vi "State Entry.vi"(8 "error in (no error)":errorcluster, 11 "View Model":T1) -> (0 "error out":errorcluster, 3 "View Model":T1)   [LabVIEW 2017]
doc: "Start processing ATM controller state when state just appear."
uses:
  View Model/Controls/View Model.ctl
  View Model/Controls/Shared Model.ctl
  Error Handler/Controls/Error Model.ctl
  Error Handler/Controls/Error Data.ctl
  Error Handler/Controls/Error Type.ctl
  Error Handler/Controls/Error Source.ctl
  Configuration/Controls/Config Model.ctl
  Configuration/Controls/Config CMD.ctl
  Configuration/Controls/Config Command.ctl
  Controls/Controller Model.ctl
  Controls/Controller Overhead.ctl
  Controls/Controller Transaction.ctl
  Controls/Controller State.ctl
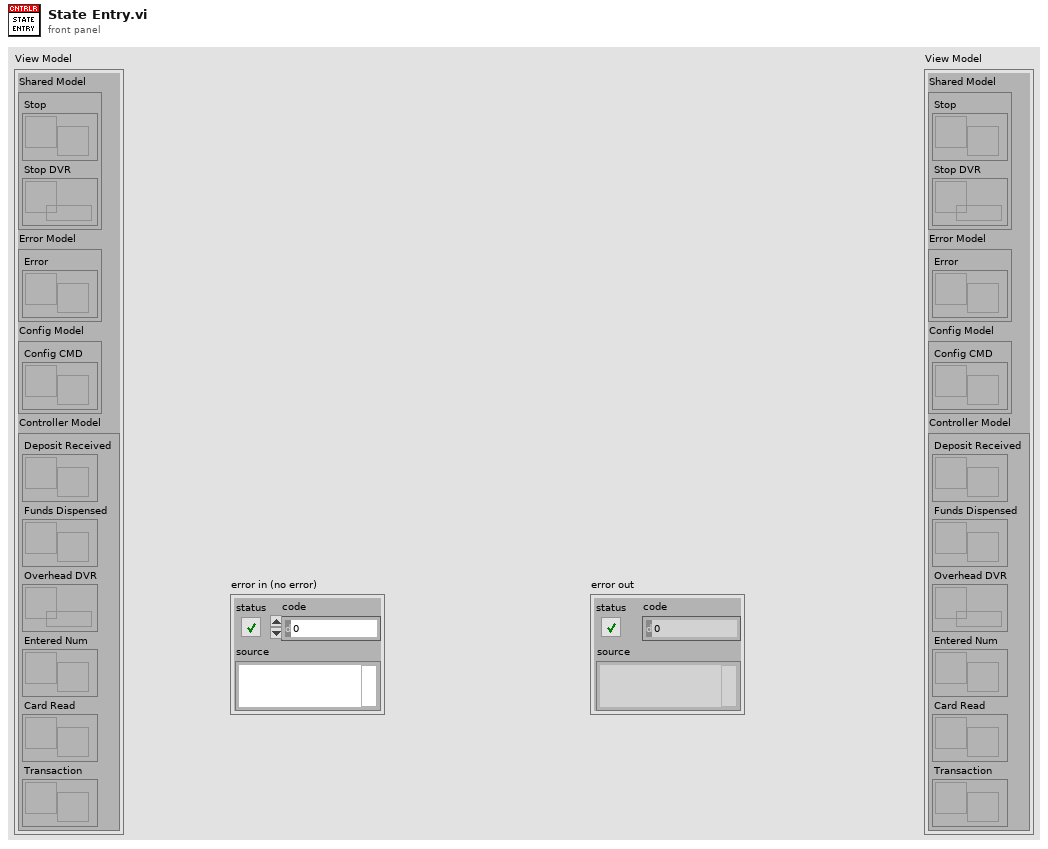
[diagram p1: front panel]
types:
  T1 = typedef "View Model.ctl" = cluster{"Shared Model":T2, "Error Model":T3, "Config Model":T4, "Controller Model":T5}
  T2 = typedef "Shared Model.ctl" = cluster{"Stop":refnum<user-event>, "Stop DVR":refnum<data-value>}
  T3 = typedef "Error Model.ctl" = cluster{"Error":refnum<user-event>}
  T4 = typedef "Config Model.ctl" = cluster{"Config CMD":refnum<user-event>}
  T5 = typedef "Controller Model.ctl" = cluster{"Deposit Received":refnum<user-event>, "Funds Dispensed":refnum<user-event>, "Overhead DVR":refnum<data-value>, "Entered Num":refnum<user-event>, "Card Read":refnum<user-event>, "Transaction":refnum<user-event>}
  T6 = typedef "Controller State.ctl" = enum16{"Idle", "Initial", "Login", "Balance Inquiry", "Deposit", "Withdrawal", "Fast Cash", "Terminate"}
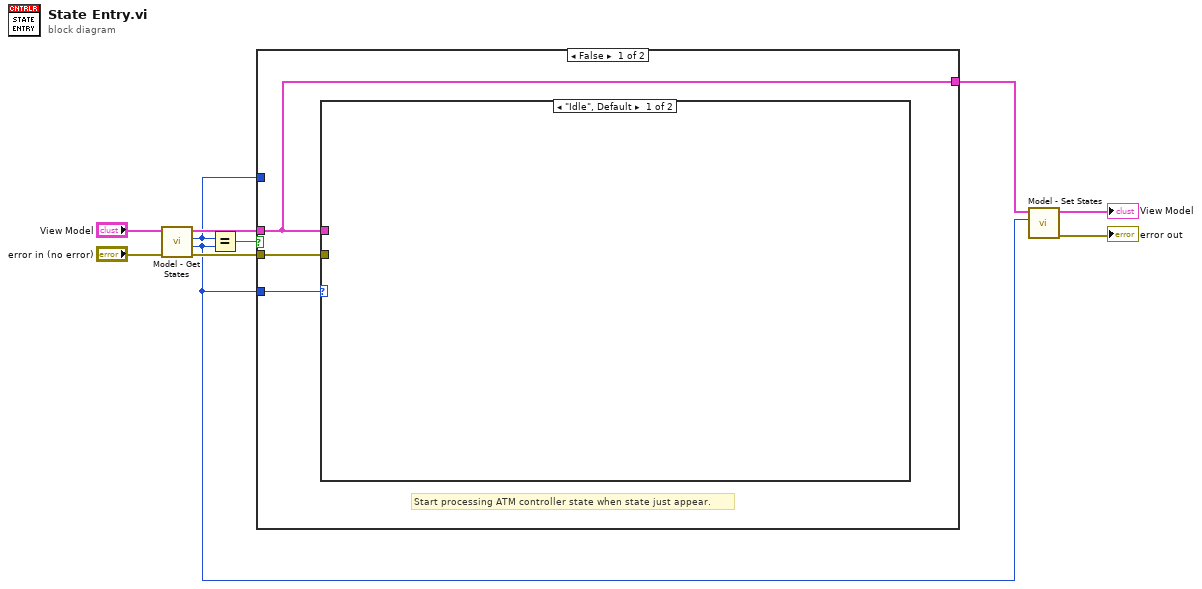
[diagram p0: block diagram]
diagram:
  n1 = call "Model - Get States.vi"("error in (no error)"="error in (no error)", "View Model"="View Model") -> ("error out"=w6:errorcluster, "Next State"=w1:T6, "Current State"=w5:T6, "View Model"=w7:T1)  [unwired: 6 in]
  n2 = Equal?(x=w5, y=w1) -> (x = y?=w8:bool)
  n3 = case shown="False" w8 {
    tunnel: w7 -> [w12 w14]
    tunnel: w6 -> [w13 _]
    tunnel: w5 -> [_ _]
    tunnel: [w12 w14] -> w4
    tunnel: w1 -> [w11 _]
    frame False {
      # "Start processing ATM controller state when state just appear."
      n4 = case shown="\"Idle\", Default" w11 {
        tunnel: w12 -> [_ _]
        tunnel: w13 -> [_ _]
        frame "Idle", Default {
        }
        frame "Initial" {
        }
      }
    }
    frame True {
    }
  }
  n5 = call "Model - Set States.vi"("Current State"=w1, "View Model"=w4) -> ("error out"=→"error out":errorcluster, "View Model"=→"View Model":T1)  [unwired: 8 in]
